vi "RC_Client.vi"(8 "error in (no error)":errorcluster, 10 "ID":i32, 11 "RemoteControl in":refnum<class "RemoteControl.lvclass">) -> (0 "error out":errorcluster)   [LabVIEW 2019, in "RemoteControl.lvlib" / "RemoteControl.lvclass"]
uses:
  RemoteControl.lvclass
  Typedefs/Message--Cluster.ctl
  b7e1e2dc-a0d6-4bbd-afea-6de24c297ea6.vi
  b7e1e2dc-a0d6-4bbd-afea-6de24c297ea6.vi/fb2b3833-d409-4f7d-9660-a91da84489f2.vi
  b7e1e2dc-a0d6-4bbd-afea-6de24c297ea6.vi/84375900-6f63-49e8-955d-29de11309d97.vi
  <vilib>/Utility/Data Type/Get Type Information.vi
  <vilib>/JDP Science/JSONtext/JSON text to Variant.vi
  <vilib>/JDP Science/JSONtext/LVClass Serializer/JSONtext LVClass Serializer.lvclass
panel:
  in  "milliseconds to wait":u32
  out "time (1 message) (s)":dbl
  out "startup time (s)":dbl
  out "messages/s":dbl
  in  "remote port":u16=6341
  in  "address":string
  out "Response":string
  out "Messages":i32
  in  "Stop":bool
  out "Command reponse":string
  out "Command":string
  out "meta data\n(available commands)":string
  # "CLIENT (API)"
  # "Connection info"
  # "Message Sent"
  # "Message Received"
  # "Metrics"
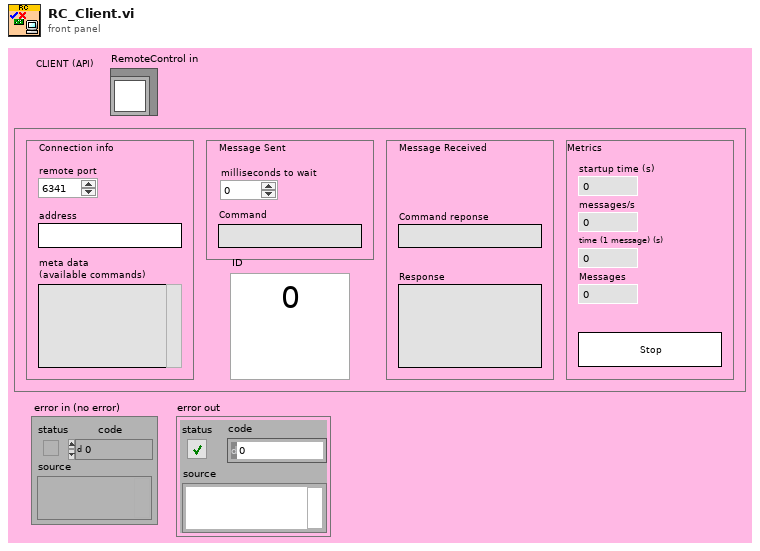
[diagram p1: front panel]
types:
  T1 = typedef "RemoteControl.lvlib/RemoteControl.lvclass/Message--Cluster.ctl" = cluster{"Command":string, "Data":variant, "ID":string, "error":errorcluster}
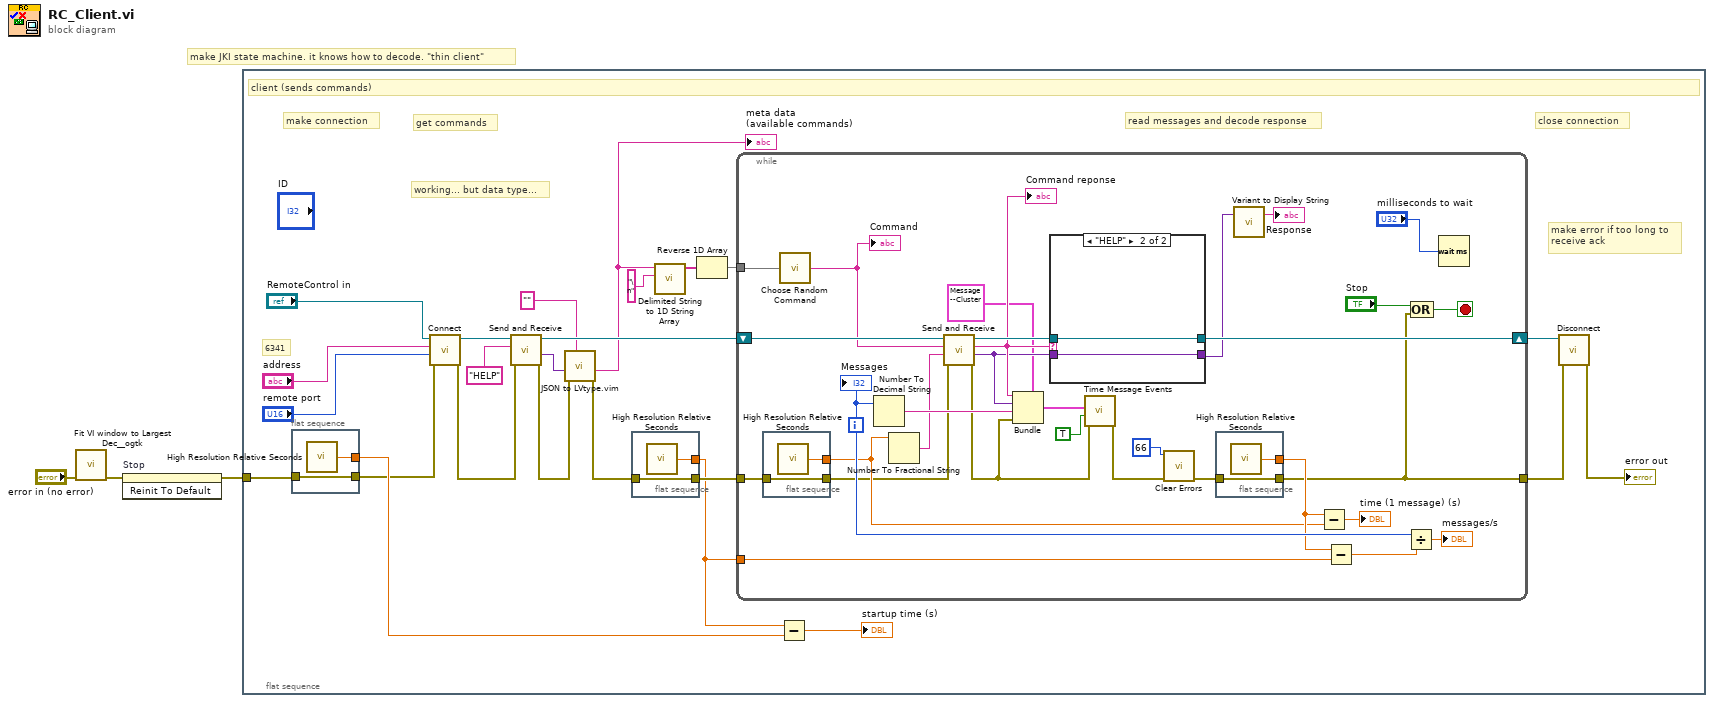
[diagram p0: block diagram]
diagram:
  # "make JKI state machine. it knows how to decode. \"thin client\""
  n1 = call <userlib>:"Fit VI window to Largest Dec__ogtk.vi"("error in (no error)"="error in (no error)") -> ("error out"=w3:errorcluster)  [unwired: 5 in, 1 out]
  n2 = invoke on="Stop" class="Bool" method="Reinit To Default"(error in=w3) -> (error out=w2:errorcluster)  [unwired: 2 in, 2 out]
  n3 = flat-sequence {
    tunnel: w2 -> [w23]
    frame #0 {
      # "working... but data type..."
      # "close connection"
      # "read messages and decode response"
      # "get commands"
      # "make connection"
      # "6341"
      # "make error if too long to\nreceive ack"
      # "client (sends commands)"
      n4 = flat-sequence {
        tunnel: [w28] -> w16
        tunnel: [w29] -> w22
        tunnel: w23 -> [w28]
        frame #0 {
          n5 = call <vilib>:"High Resolution Relative Seconds.vi"() -> ("relative seconds"=w29:dbl)
        }
      }
      n6 = call "Connect.vi"("error in (no error)"=w16, "Port"="remote port", "address"="address", "RemoteControl in"="RemoteControl in") -> ("error out"=w10:errorcluster, "RemoteControl out"=w11:refnum<class "RemoteControl.lvclass">)  [unwired: 6 in]
      n7 = call "Send and Receive.vi"("error in (no error)"=w10, "Command"="HELP", "RemoteControl in"=w11) -> ("error out"=w5:errorcluster, "Data out"=w8:variant, "RemoteControl out"=w9:refnum<class "RemoteControl.lvclass">)  [unwired: 5 in, 1 out]
      n8 = call "JSON to LVtype.vim"("type"="", "error in (no error)"=w5, "JSON Data in"=w8) -> ("error out"=w4:errorcluster, "Data out"=w6:string)  [unwired: 7 in]
      "meta data\n(available commands)" <- w6
      n9 = flat-sequence {
        tunnel: [w30] -> w26
        tunnel: [w31] -> w24
        tunnel: w4 -> [w30]
        frame #0 {
          n10 = call <vilib>:"High Resolution Relative Seconds.vi"() -> ("relative seconds"=w31:dbl)
        }
      }
      n11 = call <vilib>:"Delimited String to 1D String Array.vi"("delimiter"="\n", "delimited string"=w6) -> ("string array"=w21:string[])  [unwired: 9 in]
      n12 = Reverse 1D Array(array=w21) -> (reversed array=w27:string[])
      n13 = while {
        tunnel: [w32] -> w14
        tunnel: w26 -> [w53]
        tunnel: w27 -> [w52]
        tunnel: w24 -> [w59]
        shift-right: [w58] -> w15
        shift-left: w9 -> [w48]
        i -> [w57]
        stop <- w56 stop-if-true
        n14 = flat-sequence {
          tunnel: [w63] -> w45
          tunnel: [w64] -> w50
          tunnel: w53 -> [w63]
          frame #0 {
            n15 = call <vilib>:"High Resolution Relative Seconds.vi"() -> ("relative seconds"=w64:dbl)
          }
        }
        n16 = call "Choose Random Command.vi"("Array"=w52) -> ("String"=w47:string)
        "Command" <- w47
        n17 = Number To Decimal String(number=w57) -> (decimal integer string=w51:string)  [unwired: 1 in]
        n18 = Number To Fractional String(number=w50) -> (F-format string=w46:string)  [unwired: 3 in]
        n19 = call "Send and Receive.vi"("error in (no error)"=w45, "Data"=w46, "Command"=w47, "RemoteControl in"=w48) -> ("error out"=w39:errorcluster, "Data out"=w42:variant, "Command out"=w43:string, "RemoteControl out"=w44:refnum<class "RemoteControl.lvclass">)  [unwired: 4 in]
        "Command reponse" <- w43
        n20 = Bundle(cluster=T1 {"Command"="", "Data"=variant(string ""), "ID"="", "error"={"status"=FALSE, "code"=0, "source"=""}} ("Message in"), "Command"=w43, "Data"=w42, "ID"=w51, "error"=w39) -> (w49:T1)
        n21 = case shown="\"HELP\"" w43 {
          tunnel: [w67 w69] -> w40
          tunnel: w44 -> [w68 w70]
          tunnel: w42 -> [w67 w69]
          tunnel: [w68 w70] -> w58
          frame Default {
          }
          frame "HELP" {
          }
        }
        n22 = call "Time Message Events.vi"("error in (no error)"=w39, "Debug Mode"=TRUE, "Message in"=w49) -> ("error out"=w35:errorcluster)  [unwired: 5 in, 3 out]
        n23 = call <vilib>:"Clear Errors.vi"("error in (no error)"=w35, "specific error code to clear (0: all)"=66 ("error code")) -> ("error out"=w34:errorcluster)  [unwired: 4 in, 1 out]
        n24 = flat-sequence {
          tunnel: [w65] -> w32
          tunnel: [w66] -> w55
          tunnel: w34 -> [w65]
          frame #0 {
            n25 = call <vilib>:"High Resolution Relative Seconds.vi"() -> ("relative seconds"=w66:dbl)
          }
        }
        n26 = call "Variant to Display String.vi"("Variant"=w40) -> ("xml string"=→"Response":string)  [unwired: 2 in]
        n27 = Subtract(x=w55, y=w50) -> (x-y=→"time (1 message) (s)":dbl)
        n28 = Subtract(x=w55, y=w59) -> (x-y=w54:dbl)
        n29 = Divide(x=w57, y=w54) -> (x/y=→"messages/s":dbl)
        n30 = Compound Arithmetic op=OR("Stop", w32) -> (w56:bool)
        n31 = Wait (ms)(milliseconds to wait="milliseconds to wait") -> ()  [unwired: 1 out]
        "Messages" <- w57
      }
      n32 = Subtract(x=w24, y=w22) -> (x-y=→"startup time (s)":dbl)
      n33 = call "Disconnect.vi"("error in (no error)"=w14, "RemoteControl in"=w15) -> ("error out"=→"error out":errorcluster)  [unwired: 8 in, 1 out]
    }
  }
